vi "Write.vi"(8 "error in":errorcluster, 9 "Producer Ch":T1, 11 "Device Cluster.lvclass":refnum<class "Device Cluster.lvclass">) -> (0 "error out":errorcluster, 3 "output cluster":refnum<class "Device Cluster.lvclass">)   [LabVIEW 2023, in "Device Cluster.lvclass"]
uses:
  Device Cluster.lvclass
  6bfc6677-cd67-4f2d-afef-839dec9218ce.vi
  Producer Ch Array.ctl
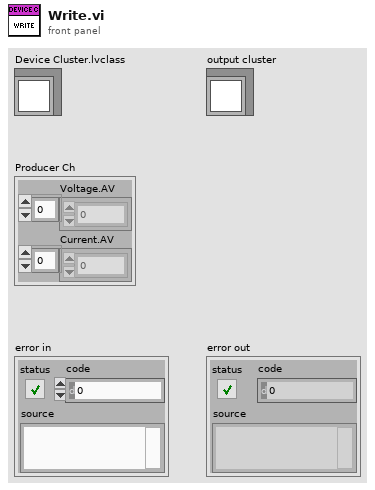
[diagram p1: front panel]
types:
  T1 = typedef "Device Cluster.lvclass/Producer Ch Array.ctl" = cluster{"Voltage.AV":dbl[], "Current.AV":dbl[]}
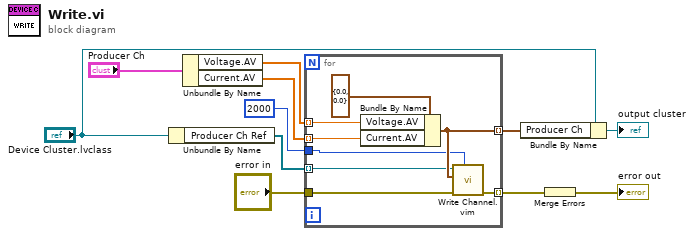
[diagram p0: block diagram]
diagram:
  n1 = Unbundle By Name("Device Cluster.lvclass") -> ("Producer Ch Ref"=w8:refnum<k21>[])
  n2 = Unbundle By Name("Producer Ch") -> ("Voltage.AV"=w2:dbl[], "Current.AV"=w1:dbl[])
  n3 = for {
    tunnel: [w19] -> w6 mode=indexing
    tunnel: "error in" -> [w18]
    tunnel: [w17] -> w4 mode=indexing
    tunnel: w8 -> [w16] mode=indexing
    tunnel: 2000 ("Timeout (ms)") -> [w15]
    tunnel: w2 -> [w13] mode=indexing
    tunnel: w1 -> [w12] mode=indexing
    n4 = Bundle By Name(cluster=cluster{"Voltage.AV":dbl, "Current.AV":dbl} {"Voltage.AV"=0.0, "Current.AV"=0.0} ("Producer Ch"), "Voltage.AV"=w13, "Current.AV"=w12) -> (w19:cluster{"Voltage.AV":dbl, "Current.AV":dbl})
    n5 = call "Write Channel.vim"("Timeout (ms)"=w15, "error in"=w18, "Data in"=w19, "ADAS HIL Channel in"=w16) -> ("error out"=w17:errorcluster)  [unwired: 5 in, 2 out]
  }
  n6 = Bundle By Name(cluster="Device Cluster.lvclass", "Producer Ch"=w6) -> (→"output cluster":refnum<class "Device Cluster.lvclass">)
  n7 = Merge Errors(w4) -> (→"error out":errorcluster)
